vi "stop.vi"(8 "error in (no error)":errorcluster, 11 "DL090202ScanHead in":refnum<class "ScanHeadDL090202.lvclass">) -> (0 "error out":errorcluster, 3 "DL090202ScanHead out":refnum<class "ScanHeadDL090202.lvclass">)   [LabVIEW 2010, in "ScanHeadDL090202.lvclass"]
uses:
  ScanHeadDL090202.lvclass
  DigitalOut/GenericDigitalOut/GenericDigitalOut/GenericDigitalOut.lvclass
  SignalWriter/GenericSignalWriter/GenericSignalWriter/GenericSignalWriter.lvclass
  Clock/GenericClock/GenericClock/GenericClock.lvclass
  common/classes/ErrorController/ErrorController/class_data.vi
  common/classes/ErrorController/ErrorController/ErrorController.lvclass
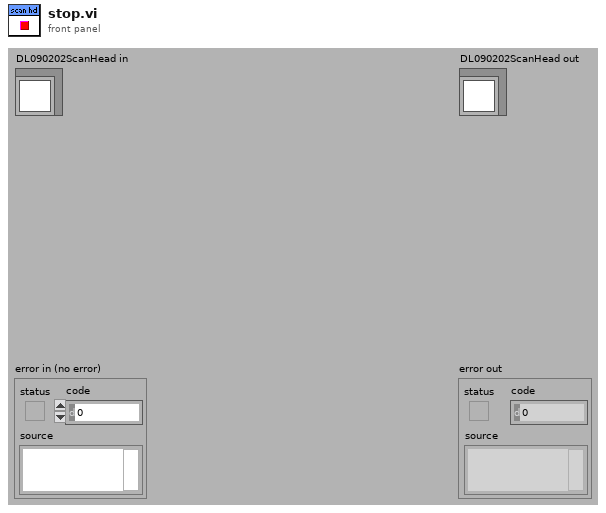
[diagram p1: front panel]
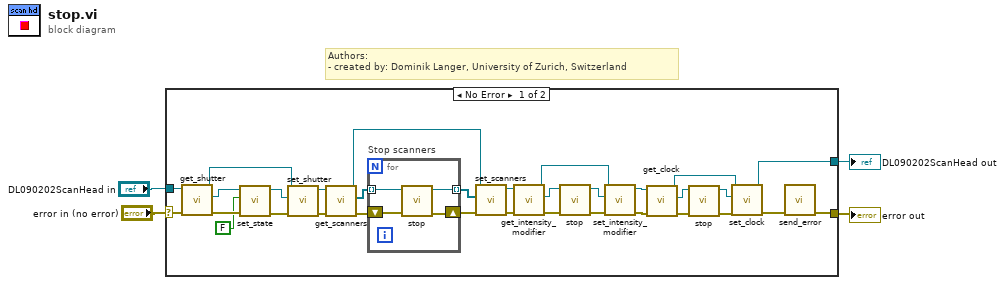
[diagram p0: block diagram]
diagram:
  # "Authors: \n- created by: Dominik Langer, University of Zurich, Switzerland"
  n1 = case shown="No Error" "error in (no error)" {
    selector: "error in (no error)" -> [w18 w42]
    tunnel: [w6 w42] -> w3
    tunnel: [w8 w41] -> w1
    tunnel: "DL090202ScanHead in" -> [w16 w41]
    frame No Error {
      n2 = call-dynamic "get_shutter.vi"("error in (no error)"=w18, "DL090202ScanHead.lvclass in"=w16) -> ("error out"=w17:errorcluster, "GenericDigitalOut.lvclass"=w15:refnum<class "GenericDigitalOut.lvclass">, "DL090202ScanHead.lvclass out"=w10:refnum<class "ScanHeadDL090202.lvclass">)  [unwired: 7 out]
      n3 = call-dynamic "set_state.vi"("error in (no error)"=w17, "state"=FALSE, "GenericDigitalOut in"=w15) -> ("error out"=w14:errorcluster, "GenericDigitalOut out"=w12:refnum<class "GenericDigitalOut.lvclass">)  [unwired: 7 in]
      n4 = call-dynamic "set_shutter.vi"("error in (no error)"=w14, "GenericDigitalOut.lvclass"=w12, "DL090202ScanHead.lvclass in"=w10) -> ("error out"=w13:errorcluster, "DL090202ScanHead.lvclass out"=w11:refnum<class "ScanHeadDL090202.lvclass">)  [unwired: 7 out]
      n5 = call-dynamic "get_scanners.vi"("error in (no error)"=w13, "DL090202ScanHead.lvclass in"=w11) -> ("error out"=w20:errorcluster, "scanners"=w21:refnum<class "GenericSignalWriter.lvclass">[], "DL090202ScanHead.lvclass out"=w19:refnum<class "ScanHeadDL090202.lvclass">)  [unwired: 7 out]
      n6 = for "Stop scanners" {
        shift-right: [w39] -> w24
        shift-left: w20 -> [w40]
        tunnel: [w38] -> w22 mode=indexing
        tunnel: w21 -> [w37] mode=indexing
        n7 = call-dynamic "stop.vi"("error in (no error)"=w40, "WriteSignalsGenericPlugin in"=w37) -> ("error out"=w39:errorcluster, "WriteSignalsGenericPlugin out"=w38:refnum<class "GenericSignalWriter.lvclass">)  [unwired: 8 out]
      }
      n8 = call-dynamic "set_scanners.vi"("error in (no error)"=w24, "scanners"=w22, "DL090202ScanHead.lvclass in"=w19) -> ("error out"=w27:errorcluster, "DL090202ScanHead.lvclass out"=w26:refnum<class "ScanHeadDL090202.lvclass">)  [unwired: 7 out]
      n9 = call-dynamic "get_intensity_modifier.vi"("error in (no error)"=w27, "DL090202ScanHead.lvclass in"=w26) -> ("error out"=w23:errorcluster, "write signals"=w25:refnum<class "GenericSignalWriter.lvclass">, "DL090202ScanHead.lvclass out"=w9:refnum<class "ScanHeadDL090202.lvclass">)  [unwired: 7 out]
      n10 = call-dynamic "stop.vi"("error in (no error)"=w23, "WriteSignalsGenericPlugin in"=w25) -> ("error out"=w35:errorcluster, "WriteSignalsGenericPlugin out"=w36:refnum<class "GenericSignalWriter.lvclass">)  [unwired: 8 out]
      n11 = call-dynamic "set_intensity_modifier.vi"("error in (no error)"=w35, "write signals"=w36, "DL090202ScanHead.lvclass in"=w9) -> ("error out"=w34:errorcluster, "DL090202ScanHead.lvclass out"=w28:refnum<class "ScanHeadDL090202.lvclass">)  [unwired: 7 out]
      n12 = call-dynamic "get_clock.vi"("error in (no error)"=w34, "DL090202ScanHead.lvclass in"=w28) -> ("error out"=w33:errorcluster, "GenericClock.lvclass"=w32:refnum<class "GenericClock.lvclass">, "DL090202ScanHead.lvclass out"=w29:refnum<class "ScanHeadDL090202.lvclass">)  [unwired: 7 out]
      n13 = call-dynamic "stop.vi"("error in (no error)"=w33, "GenericClock in"=w32) -> ("error out"=w31:errorcluster, "GenericClock out"=w30:refnum<class "GenericClock.lvclass">)  [unwired: 8 out]
      n14 = call-dynamic "set_clock.vi"("error in (no error)"=w31, "GenericClock.lvclass"=w30, "DL090202ScanHead.lvclass in"=w29) -> ("error out"=w7:errorcluster, "DL090202ScanHead.lvclass out"=w8:refnum<class "ScanHeadDL090202.lvclass">)  [unwired: 7 out]
      n15 = call "send_error.vi"("error in (no error)"=w7) -> ("error out"=w6:errorcluster)  [unwired: 10 in]
    }
    frame Error {
    }
  }
  "error out" <- w3
  "DL090202ScanHead out" <- w1
